vi "Initiate.vi"(8 "error in (no error)":errorcluster, 11 "VISA resource name":refnum<visa-resource-name>) -> (0 "error out":errorcluster, 3 "VISA resource name out":refnum<visa-resource-name>)   [LabVIEW 2018, in "Agilent MXA Series.lvlib"]
doc: "Initiates a trace sweep. After you call this VI, the instrument leaves the idle state and waits for a trigger.\n\n<B>Note:</B>\n\nUse this VI only with other low-level VIs. The high-level VIs automatically incorporate this functionality. This VI does not check the instrument status."
uses:
  Agilent MXA Series.lvlib
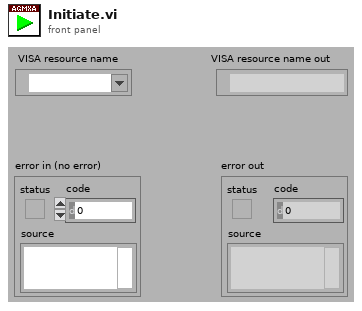
[diagram p1: front panel]
types:
  T1 = typedef "Agilent MXA Series.lvlib/Extended User Data.ctl" = cluster{"Measurement Type":i32, "Agilent MXA/EXA Model":i32}
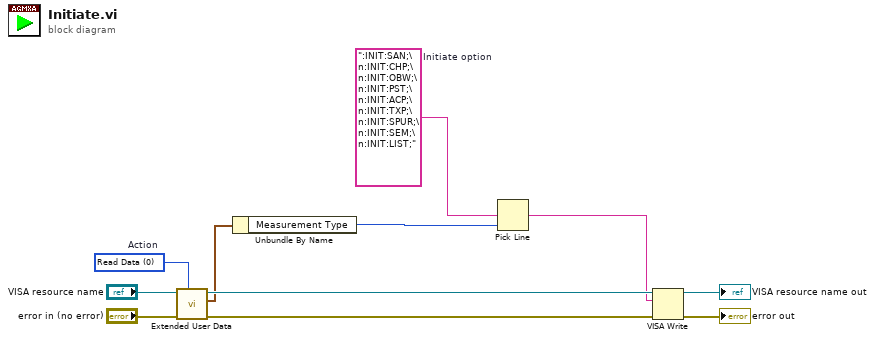
[diagram p0: block diagram]
diagram:
  w2 = ":INIT:SAN;\n:INIT:CHP;\n:INIT:OBW;\n:INIT:PST;\n:INIT:ACP;\n:INIT:TXP;\n:INIT:SPUR;\n:INIT:SEM;\n:INIT:LIST;"  # Initiate option
  w5 = 0 items=["Read Data", "Write Data", "Clear Data", "Clear ALL Data"]  # Action
  n1 = call "Extended User Data.vi"("Action (1:Write Data)"=w5, "Error In (no error)"="error in (no error)", "VISA resource name in"="VISA resource name") -> ("Error Out"=w6:errorcluster, "User Data Out"=w4:T1, "VISA resource name out"=w7:refnum<visa-resource-name>)  [unwired: 6 in]
  n2 = Unbundle By Name(w4) -> ("Measurement Type"=w3:i32)
  n3 = Pick Line(multi-line string=w2, line index=w3) -> (output string=w1:string)  [unwired: 1 in]
  n4 = VISA Write(VISA resource name=w7, write buffer=w1, error in (no error)=w6) -> (VISA resource name out=→"VISA resource name out":refnum<visa-resource-name>, error out=→"error out":errorcluster)  [unwired: 1 out]
